vi "p8.8.vi"() -> ()   [LabVIEW 2020]
uses:
  <vilib>/vision/NI_Vision_Development_Module.lvlib
panel:
  out "IFFT":T1(plugin-control)
  out "FFT":T1(plugin-control)
  out "Imagen1":T1(plugin-control)
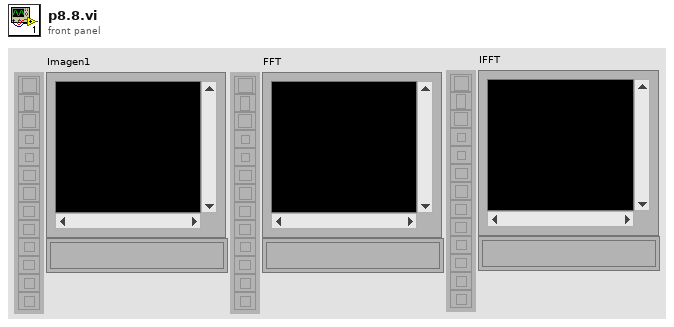
[diagram p1: front panel]
types:
  T1 = typedef "IMAQ Image.ctl" = refnum<image>
  T2 = typedef "Image Type" = u32
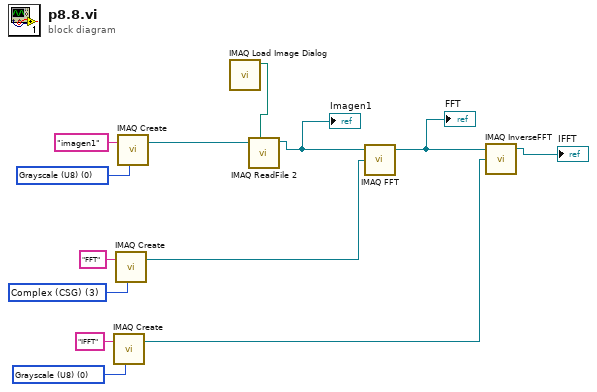
[diagram p0: block diagram]
diagram:
  w1 = T2 0 items=["Grayscale (U8)", "Grayscale (I16)", "Grayscale (SGL)", "Complex (CSG)", "RGB (U32)", "HSL (U32)", "RGB (U64)", "Grayscale (U16)"] ("Image Type")
  w2 = T2 3 items=["Grayscale (U8)", "Grayscale (I16)", "Grayscale (SGL)", "Complex (CSG)", "RGB (U32)", "HSL (U32)", "RGB (U64)", "Grayscale (U16)"] ("Image Type")
  w3 = T2 0 items=["Grayscale (U8)", "Grayscale (I16)", "Grayscale (SGL)", "Complex (CSG)", "RGB (U32)", "HSL (U32)", "RGB (U64)", "Grayscale (U16)"] ("Image Type")
  n1 = call "IMAQ Create"("Image Name"="IFFT", "Image Type"=w1) -> ("New Image"=w7:T1)  [unwired: 3 in, 1 out]
  n2 = call "IMAQ Create"("Image Name"="FFT", "Image Type"=w2) -> ("New Image"=w9:T1)  [unwired: 3 in, 1 out]
  n3 = call "IMAQ Create"("Image Name"="imagen1", "Image Type"=w3) -> ("New Image"=w13:T1)  [unwired: 3 in, 1 out]
  n4 = call "IMAQ Load Image Dialog"() -> ("Path"=w12:path)  [unwired: 9 in, 2 out]
  n5 = call "IMAQ ReadFile 2"("File Path"=w12, "Image"=w13) -> ("Image Out"=w6:T1)  [unwired: 5 in, 4 out]
  "Imagen1" <- w6
  n6 = call "IMAQ FFT"("Image Dst"=w9, "Image Src"=w6) -> ("Image Dst Out"=w5:T1)  [unwired: 2 in, 1 out]
  "FFT" <- w5
  n7 = call "IMAQ InverseFFT"("Image Dst"=w7, "Image Src"=w5) -> ("Image Dst Out"=→"IFFT":T1)  [unwired: 2 in, 1 out]
